vi "NF87XX.ProcEvents.vi"(0 "i ref in":refnum<vi>, 5 "error in":errorcluster) -> (14 "i ref out":refnum<vi>, 19 "error out":errorcluster)   [LabVIEW 2014, in "NF87XX.lvlib"]
doc: "This method is used to define the events the object will listen to. Add your own events here."
uses:
  NF87XX.lvlib
  CS_Core/BaseProcess/BaseProcess.event definition.ctl
  CS_Core/CAEObj/CAEObj.event definition.ctl
  CS_Core/BaseProcess/BaseProcess.descriptor string definition.ctl
  CS_Core/BaseProcess/BaseProcess.lvlib
  CS_Core/CAEObj/CAEObj.lvlib
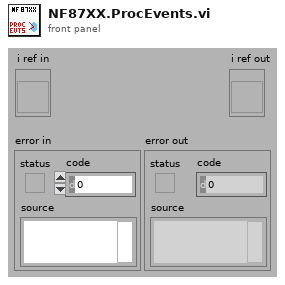
[diagram p1: front panel]
types:
  T1 = typedef "BaseProcess.lvlib/BaseProcess.event definition.ctl" = cluster{"CAEEvtDef":T2, "Data Descriptor":T3}
  T2 = typedef "CAEObj.lvlib/CAEObj.event definition.ctl" = cluster{"URL":string, "enable":bool, "ignoreResID":bool}
  T3 = typedef "BaseProcess.lvlib/BaseProcess.descriptor string definition.ctl" = string
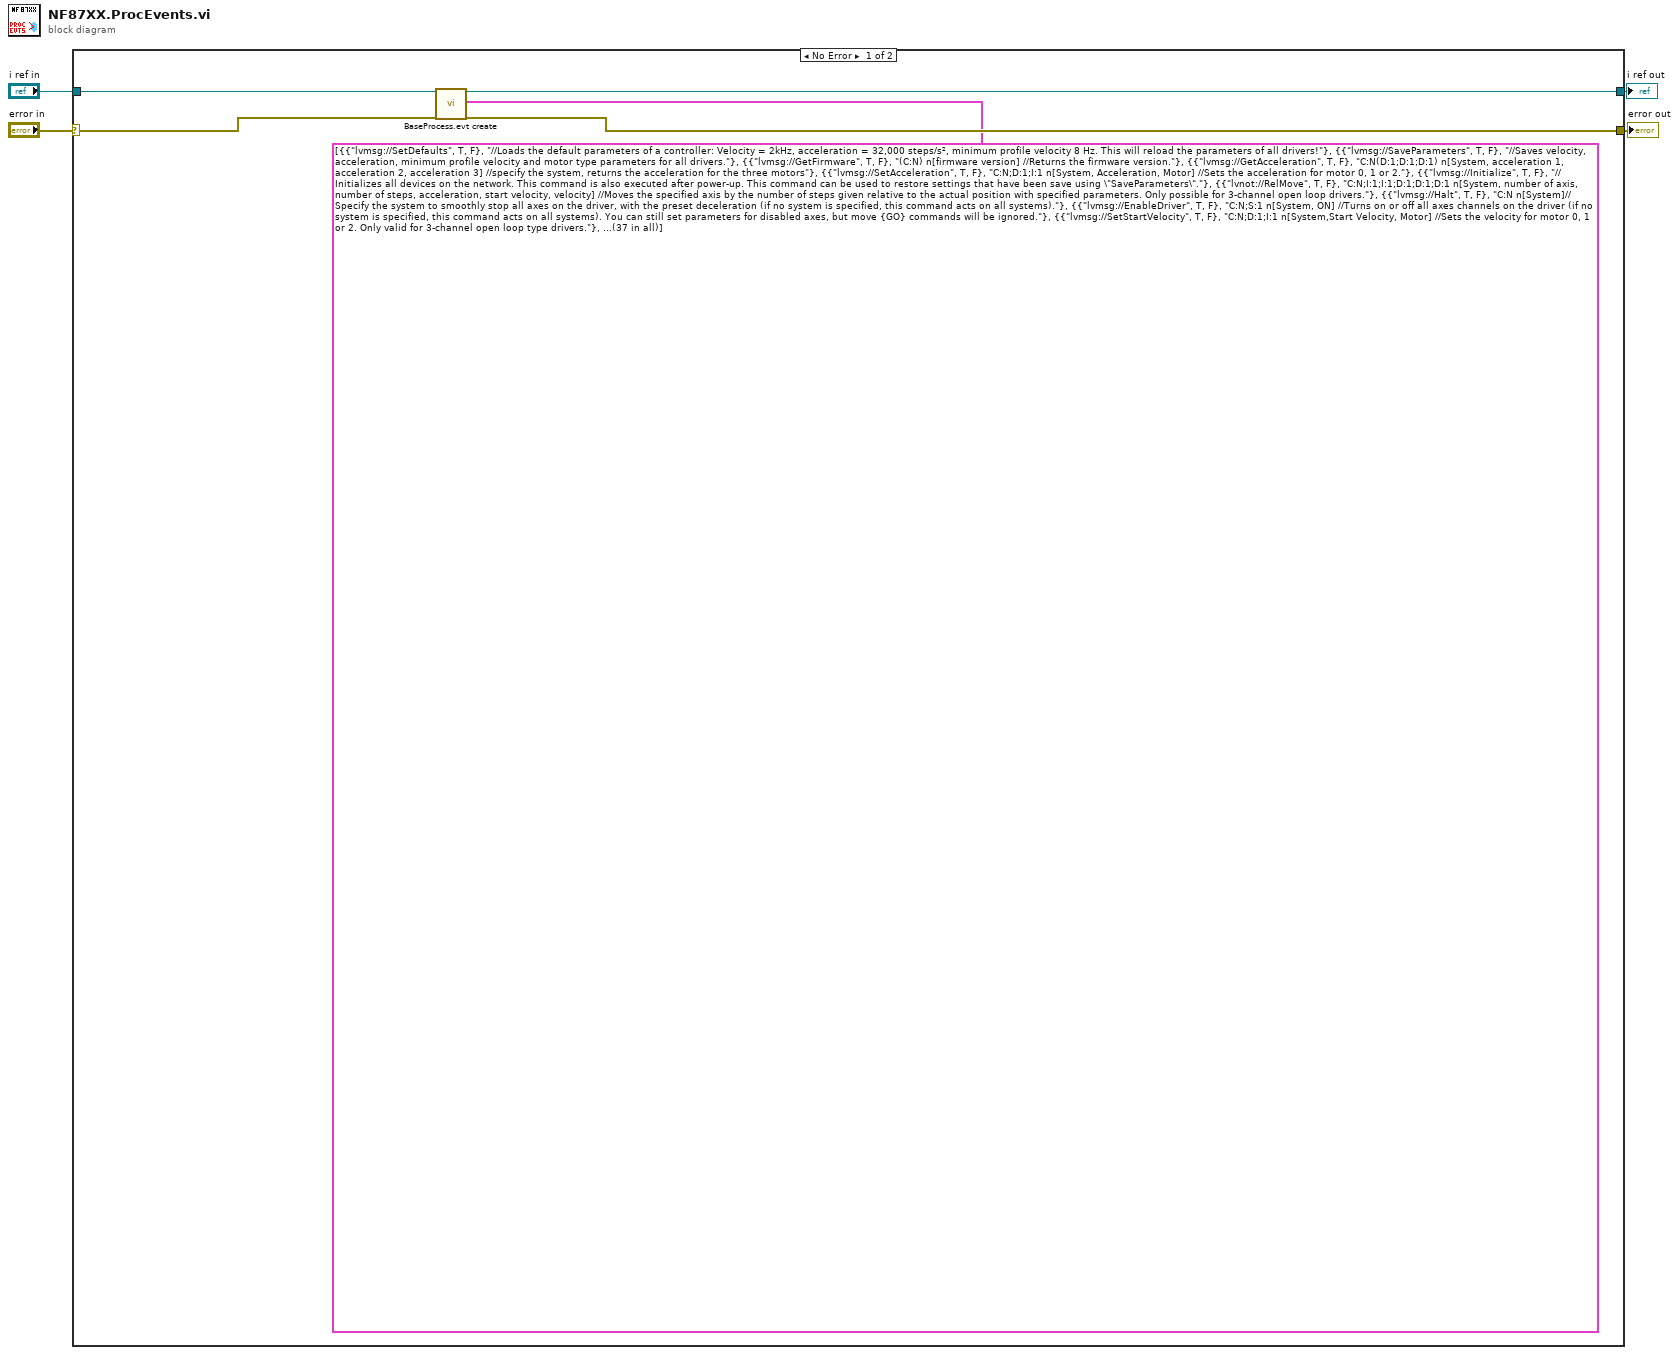
[diagram p0: block diagram]
diagram:
  n1 = case shown="No Error" "error in" {
    selector: "error in" -> [w5 w10]
    tunnel: "i ref in" -> [w9 w11]
    tunnel: [w8 w11] -> w3
    tunnel: [w7 w10] -> w2
    frame No Error {
      n2 = call "BaseProcess.evt create.vi"("i ref in"=w9, "newEvents"=T1[] [{"CAEEvtDef"={"URL"="lvmsg://SetDefaults", "enable"=TRUE, "ignoreResID"=FALSE}, "Data Descriptor"="//Loads the default parameters of a controller: Velocity = 2kHz, acceleration = 32,000 steps/s², minimum profile velocity 8 Hz. This will reload the parameters of all drivers!"}, {"CAEEvtDef"={"URL"="lvmsg://SaveParameters", "enable"=TRUE, "ignoreResID"=FALSE}, "Data Descriptor"="//Saves velocity, acceleration, minimum profile velocity and motor type parameters for all drivers."}, {"CAEEvtDef"={"URL"="lvmsg://GetFirmware", "enable"=TRUE, "ignoreResID"=FALSE}, "Data Descriptor"="(C:N) n[firmware version] //Returns the firmware version."}, {"CAEEvtDef"={"URL"="lvmsg://GetAcceleration", "enable"=TRUE, "ignoreResID"=FALSE}, "Data Descriptor"="C:N(D:1;D:1;D:1) n[System, acceleration 1, acceleration 2, acceleration 3] //specify the system, returns the acceleration for the three motors"}, {"CAEEvtDef"={"URL"="lvmsg://SetAcceleration", "enable"=TRUE, "ignoreResID"=FALSE}, "Data Descriptor"="C:N;D:1;I:1 n[System, Acceleration, Motor] //Sets the acceleration for motor 0, 1 or 2."}, {"CAEEvtDef"={"URL"="lvmsg://Initialize", "enable"=TRUE, "ignoreResID"=FALSE}, "Data Descriptor"="//Initializes all devices on the network. This command is also executed after power-up. This command can be used to restore settings that have been save using \"SaveParameters\"."}, {"CAEEvtDef"={"URL"="lvnot://RelMove", "enable"=TRUE, "ignoreResID"=FALSE}, "Data Descriptor"="C:N;I:1;I:1;D:1;D:1;D:1 n[System, number of axis, number of steps, acceleration, start velocity, velocity] //Moves the specified axis by the number of steps given relative to the actual position with specified parameters. Only possible for 3-channel open loop drivers."}, {"CAEEvtDef"={"URL"="lvmsg://Halt", "enable"=TRUE, "ignoreResID"=FALSE}, "Data Descriptor"="C:N n[System]//Specify the system to smoothly stop all axes on the driver, with the preset deceleration (if no system is specified, this command acts on all systems)."}, {"CAEEvtDef"={"URL"="lvmsg://EnableDriver", "enable"=TRUE, "ignoreResID"=FALSE}, "Data Descriptor"="C:N;S:1 n[System, ON] //Turns on or off all axes channels on the driver (if no system is specified, this command acts on all systems). You can still set parameters for disabled axes, but move {GO} commands will be ignored."}, {"CAEEvtDef"={"URL"="lvmsg://SetStartVelocity", "enable"=TRUE, "ignoreResID"=FALSE}, "Data Descriptor"="C:N;D:1;I:1 n[System,Start Velocity, Motor] //Sets the velocity for motor 0, 1 or 2. Only valid for 3-channel open loop type drivers."}, {"CAEEvtDef"={"URL"="lvmsg://GetStartVelocity", "enable"=TRUE, "ignoreResID"=FALSE}, "Data Descriptor"="C:N(D:1;D:1;D:1) n[system, start velocity 0, start velocity 1, start velocity 2] //specify the system, returns the \"start velocity\" {miminum of a velocity profile} in steps/s for the three motors. Only valid for 3-channel open loop type drivers."}, {"CAEEvtDef"={"URL"="lvmsg://GetStatus", "enable"=TRUE, "ignoreResID"=FALSE}, "Data Descriptor"="(C:N) n[status] //Returns the status of the driver."}, {"CAEEvtDef"={"URL"="lvmsg://Stop", "enable"=TRUE, "ignoreResID"=FALSE}, "Data Descriptor"="C:N n[System]//Abruptly stops the motion of active axes of the system (if no system is specified, this command acts on all systems). "}, {"CAEEvtDef"={"URL"="lvmsg://GetVelocity", "enable"=TRUE, "ignoreResID"=FALSE}, "Data Descriptor"="C:N(D:1;D:1;D:1) n[system,velocity 1, velocity 2, velocity 3] //specify the system, returns the velocity in velocity mode or stop velocity in trapezoidal mode {steps/s} for all three motors."}, {"CAEEvtDef"={"URL"="lvmsg://SetVelocity", "enable"=TRUE, "ignoreResID"=FALSE}, "Data Descriptor"="C:N;D:1;I:1 n[System, Velocity, Motor] //Sets the velocity for motor 0, 1 or 2."}, {"CAEEvtDef"={"URL"="lvmsg://Reset", "enable"=TRUE, "ignoreResID"=FALSE}, "Data Descriptor"="//Resets the systems as well as the controller: This method has side effects on other drivers attached to the same controller. This method restores the previously saved parameters and enables the driver.\n"}, {"CAEEvtDef"={"URL"="lvmsg://LockInputDevice", "enable"=TRUE, "ignoreResID"=FALSE}, "Data Descriptor"="//Locks out all other connected input devices."}, {"CAEEvtDef"={"URL"="lvmsg://UnLockInputDevice", "enable"=TRUE, "ignoreResID"=FALSE}, "Data Descriptor"="//Removes locks against other connected input devices."}, {"CAEEvtDef"={"URL"="lvmsg://GetDriverType", "enable"=TRUE, "ignoreResID"=FALSE}, "Data Descriptor"="(S:N) n[driver types] //Returns the driver types in the order of the systems: \"0\" for no information, \"1\" for 3-channel open -, \"2\" for 1-channel closed loop driver."}, {"CAEEvtDef"={"URL"="lvmsg://Start", "enable"=TRUE, "ignoreResID"=FALSE}, "Data Descriptor"="C:N n[System]//Starts all axes of the system with the current configuration."}, {"CAEEvtDef"={"URL"="lvmsg://GetMotorType", "enable"=TRUE, "ignoreResID"=FALSE}, "Data Descriptor"="C:N;I:1(S:1) n[System, Motor, Motor Type] //Returns the configured motor type which is either \"0\" (standard picomotor) or \"1\" (tiny picomotor). \"2\" indicates \"no information\""}, {"CAEEvtDef"={"URL"="lvmsg://SetMotorType", "enable"=TRUE, "ignoreResID"=FALSE}, "Data Descriptor"="C:N;S:1;I:1 n[System, Motor Type, Motor] //Configures the motor type; \"0\" (standard picomotor) or \"1\" (tiny picomotor)."}, {"CAEEvtDef"={"URL"="lvmsg://EnableJoystick", "enable"=TRUE, "ignoreResID"=FALSE}, "Data Descriptor"="S:1 n[ON] //Turns on or off the joystick."}, {"CAEEvtDef"={"URL"="lvmsg://GetChannel", "enable"=TRUE, "ignoreResID"=FALSE}, "Data Descriptor"="C:N(I:1) n[System, Channel]//specify the system, returns the active channel. Only valid for 3-channel open loop type drivers."}, {"CAEEvtDef"={"URL"="lvmsg://SetChannel", "enable"=TRUE, "ignoreResID"=FALSE}, "Data Descriptor"="C:N;I:1 n[System,Channel]//Sets the systems, selects the active motor channel, must be 0, 1 or 2. Only valid for 3-channel open loop type drivers."}, {"CAEEvtDef"={"URL"="lvmsg://SetRelPosition", "enable"=TRUE, "ignoreResID"=FALSE}, "Data Descriptor"="C:N;I:1;S:1 n[System,Steps, Immediately?]//Sets the amount of steps to move for the specified system. If true is chosen, movement start immediately."}, {"CAEEvtDef"={"URL"="lvmsg://GetMacAddress", "enable"=TRUE, "ignoreResID"=FALSE}, "Data Descriptor"="(C:N) n[MAC Address]// Gets the MAC address of the device."}, {"CAEEvtDef"={"URL"="lvmsg://GetHostname", "enable"=TRUE, "ignoreResID"=FALSE}, "Data Descriptor"="(C:N) n[Hostname]// Gets the Hostname."}, {"CAEEvtDef"={"URL"="lvmsg://SetAbsPosition", "enable"=TRUE, "ignoreResID"=FALSE}, "Data Descriptor"="C:N;I:1;S:1 n[System, Position, Immediately?]//Specify the system, sets the position to go to. If true is chosen, movement start immediately."}, {"CAEEvtDef"={"URL"="lvmsg://FindIndexMark", "enable"=TRUE, "ignoreResID"=FALSE}, "Data Descriptor"="C:N;S:1 n[System, forward?]//Specify the system, move forward (true) or backward (false) to the index mark (middle position)."}, {"CAEEvtDef"={"URL"="lvmsg://FindLimit", "enable"=TRUE, "ignoreResID"=FALSE}, "Data Descriptor"="C:N;S:1 n[System, forward?]//Specify the system, move to forward limit (true) or backward limit (false)."}, {"CAEEvtDef"={"URL"="lvmsg://SetLoopMode", "enable"=TRUE, "ignoreResID"=FALSE}, "Data Descriptor"="S:1 n[closed loop on]//Turns the closed loop mode on or off. Only valid for 1-channel closed loop type drivers."}, {"CAEEvtDef"={"URL"="lvmsg://GetPosition", "enable"=TRUE, "ignoreResID"=FALSE}, "Data Descriptor"="//In case of a closed loop system, the positions are figured out and pblished via DIM service."}, {"CAEEvtDef"={"URL"="lvmsg://SetPosition", "enable"=TRUE, "ignoreResID"=FALSE}, "Data Descriptor"="C:N;I:1 n[System, Position]//Sets the position of the specified system if this is closed loop type."}, {"CAEEvtDef"={"URL"="lvnot://AbsMove", "enable"=TRUE, "ignoreResID"=FALSE}, "Data Descriptor"="C:N;S:1;D:1 n[System, forward?, Velocity]//Sets the velocity of the selected system and starts the move to the absolute position. Only possible for 1-channel closed loop drivers."}, {"CAEEvtDef"={"URL"="lvmsg://SetFineSpeed", "enable"=TRUE, "ignoreResID"=FALSE}, "Data Descriptor"="//sets the velocity to fine (250Hz) speed"}, {"CAEEvtDef"={"URL"="lvmsg://SetCoarseSpeed", "enable"=TRUE, "ignoreResID"=FALSE}, "Data Descriptor"="//sets the velocity to coarse (2000Hz) speed"}] ("new events(V3.0)"), "error in (no error)"=w5) -> ("i ref out"=w8:refnum<vi>, "error out"=w7:errorcluster)  [unwired: 13 in, 2 out]
    }
    frame Error {
    }
  }
  "i ref out" <- w3
  "error out" <- w2
